vi "Auto Encoder Steering.vi"(8 "Backward":bool, 9 "Gyro Angle":dbl, 11 "Angle setpoint":dbl) -> (1 "Steering":dbl, 3 "Angle error":dbl)   [LabVIEW 2013]
uses:
  Robot Global Data.vi
  <vilib>/addons/control/pid/pid.llb/PID (DBL).vi
  <vilib>/addons/control/pid/NI_PID_pid.lvlib
panel:
  in  "Auto/Control/Steer Limit":dbl=0.7 caption="Turning Limit"
  out "Auto/Output/Gyro Error":dbl caption="Output"
  in  "Auto/Control/Drift Correction Backward Gryo":dbl=0.08 caption="Steering Power"
  in  "Auto/Control/Drift Correction Forward Gryo":dbl=-0.08 caption="Steering Power"
  in  "Auto/Control/Drift Correction Backward":dbl=0.007 caption="Steering Power"
  in  "Auto/Control/Gryo Steering":bool=TRUE caption="Gryo Steering"
  out "Auto/Output/Steering":dbl caption="Output"
  in  "Auto/Control/Drift Correction Forward":dbl=0.007 caption="Steering Power"
  out "Auto/Output/Encoder Error":dbl caption="Output"
  out "Steering Output Graph":dbl(graph)
  in  "Left Dist":dbl
  in  "Right Dist":dbl
  out "Error":dbl(graph)
  # "Steering Power"
  # "Encoder"
  # "Gyro"
  # "Error"
  # "Forward"
  # "Backward"
  # "Drive X-Axis power\nper 1 encoder unit\ndifference L/R"
  # "DISABLED -->"
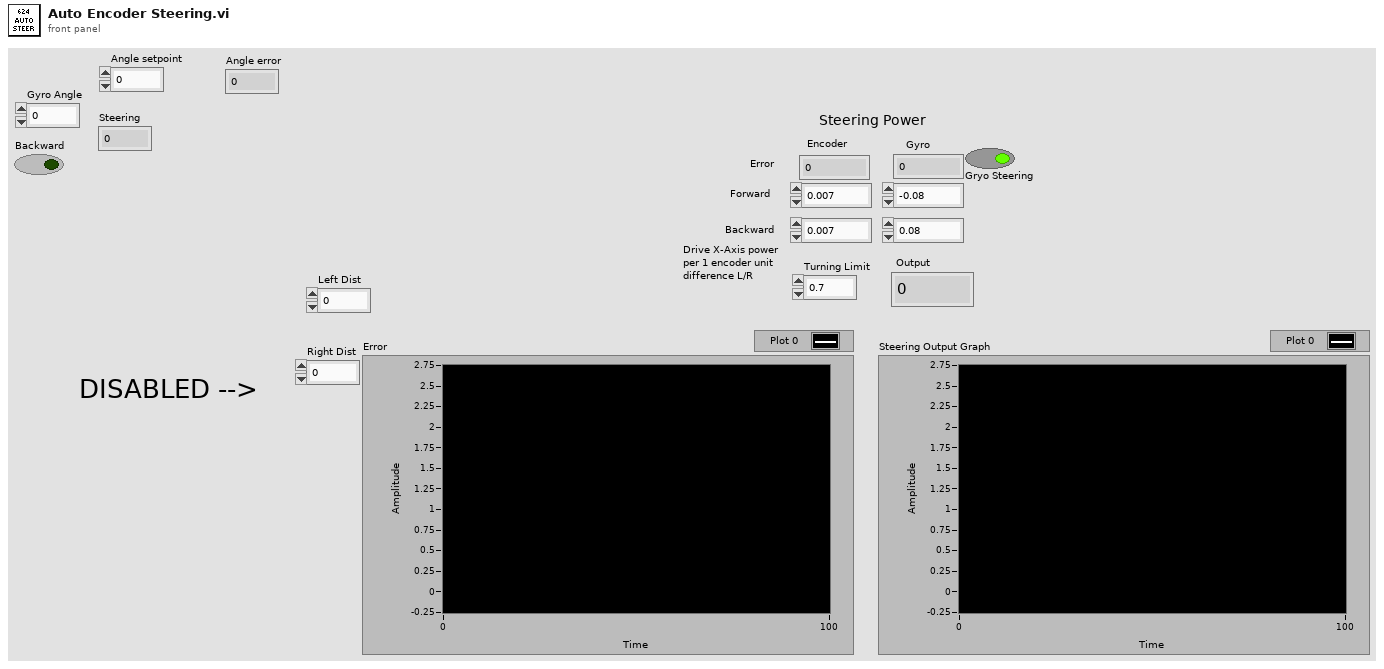
[diagram p1: front panel]
types:
  T1 = typedef "Encoder Values.ctl" = cluster{"Left Dist":dbl, "Left Speed":dbl, "Right Dist":dbl, "Right Speed":dbl, "Left Ticks":dbl, "Right Ticks":dbl, "Avg Distance":dbl, "Avg Speed":dbl}
  T2 = typedef "UDP Dashboard Packet.ctl" = cluster{"Feed Angle":dbl, "Neutral Angle":dbl, "Autonomous Setpoints":T3, "Auto Shift":T4, "Elevator Angle Offset":dbl, "Potentiometer Angle":cluster{"Pot M":dbl, "Pot B":dbl}, "Shoot Setpoints":cluster{"Vision":T5, "Back Corner":T5, "Front":T5, "Front Corner":T5, "Half Court":T5, "Full Court":T5, "Pyramid":T5}, "Halo Drive":T6, "Auto Speed Constants":T7, "Shooting Delays":cluster{"Unjam On":dbl, "Unjam Off":dbl, "Flipper On":dbl, "Flipper Off":dbl, "Hopper Up":dbl}, "Left Roller Pwr":dbl, "Right Roller Pwr":dbl, "Elevator PID Gains":cluster{"proportional gain (Kc)":dbl, "integral time (Ti, min)":dbl, "derivative time (Td, min)":dbl}, "Elevator PID Output Range":cluster{"output high":dbl, "output low":dbl}, "Elevator Angle Tolerance":dbl, "Toggle Ears Delay":dbl, "Toggle Ears Distance":dbl, "Unjam Servo Angle":dbl, "Auton Steer PID gains":cluster{"proportional gain (Kc)":dbl, "integral time (Ti, min)":dbl, "derivative time (Td, min)":dbl}, "Auton Steer output range":cluster{"output high":dbl, "output low":dbl}, "Auto Reverse Speed":dbl, "Auto Stop Throttle":dbl, "Auto Stop Duration":dbl, "Spin output range":cluster{"output high":dbl, "output low":dbl}, "Spin PID gains":cluster{"proportional gain (Kc)":dbl, "integral time (Ti, min)":dbl, "derivative time (Td, min)":dbl}, "Auto-Center Line":T8, "Auton Distance PID gains Low Gear":cluster{"proportional gain (Kc)":dbl, "integral time (Ti, min)":dbl, "derivative time (Td, min)":dbl}, "Auton Distance output range":cluster{"output high":dbl, "output low":dbl}, "Auton Distance Threshold":dbl, "Auton Velocity Cutoff":dbl, "Auton Distance output range Center Line":cluster{"output high":dbl, "output low":dbl}, "Auton Distance PID gains High Gear":cluster{"proportional gain (Kc)":dbl, "integral time (Ti, min)":dbl, "derivative time (Td, min)":dbl}}
  T3 = typedef "Autonomous Setpoints.ctl" = cluster{"Shoot Angle 1":dbl, "Initial Delay":dbl, "Disc Count 1":dbl, "Shoot Time 1":dbl, "Distance 1":dbl, "Two Disc Distance 1":dbl, "Distance 2":dbl, "Two Disc Distance 2":dbl, "Distance 3":dbl, "Two Disc Distance 3":dbl, "Shoot Angle 3":dbl, "Disc Count 3":dbl, "Shoot Time 3":dbl, "Distance 4":dbl, "Two Disc Distance 4":dbl, "Low Gear":bool, "Shoot 1 Post Delay":dbl}
  T4 = typedef "Auto Shift Settings.ctl" = cluster{"Enabled":bool, "Upshift Speed":dbl, "Downshift Speed":dbl, "Upshift Throttle":dbl, "Turn Power Diff":dbl, "Motor Limit":dbl, "Encoder Limit":dbl}
  T5 = typedef "Shoot Profile.ctl" = cluster{"Pre RPM":dbl, "Main RPM":dbl, "Angle":dbl}
  T6 = typedef "Halo Drive.ctl" = cluster{"Gains":cluster{"Quickturn_Sens_Low":dbl, "Quickturn_Sens_High":dbl, "Speedturn_Sens_Low":dbl, "Speedturn_Sens_High":dbl}, "QuickTurn Const":dbl, "Loading Throttle Limit":dbl}
  T7 = typedef "Auto Speed Constants.ctl" = cluster{"Slowing Distance":dbl, "High Speed":dbl, "Rampup Time":dbl, "Low Speed":dbl, "High Speed (Reverse)":dbl}
  T8 = typedef "Autonomous Center Line Setpoints.ctl" = cluster{"Arc Turn x-axis":dbl, "Arc Turn y-axis":dbl, "Arc Turn Distance":dbl, "Distance 1":dbl, "Two Disc Distance 1":dbl, "Distance 2":dbl, "Two Disc Distance 2":dbl, "Spin Angle":dbl, "Spin Angle tolerance":dbl, "Spin y-axis":dbl, "Spin Distance":dbl, "Center Line Enabled":bool, "Distance 3":dbl, "Two Disc Distance 3":dbl, "Spin Angle 2":dbl, "Spin Angle tolerance 2":dbl, "Spin y-axis 2":dbl, "Spin Distance 2":dbl, "Shoot Angle 1":dbl, "Disc Count 1":dbl, "Shoot Time 1":dbl, "Shoot Angle 3":dbl, "Disc Count 3":dbl, "Shoot Time 3":dbl, "Low Gear":bool}
  T9 = cluster{"proportional gain (Kc)":dbl, "integral time (Ti, min)":dbl, "derivative time (Td, min)":dbl}
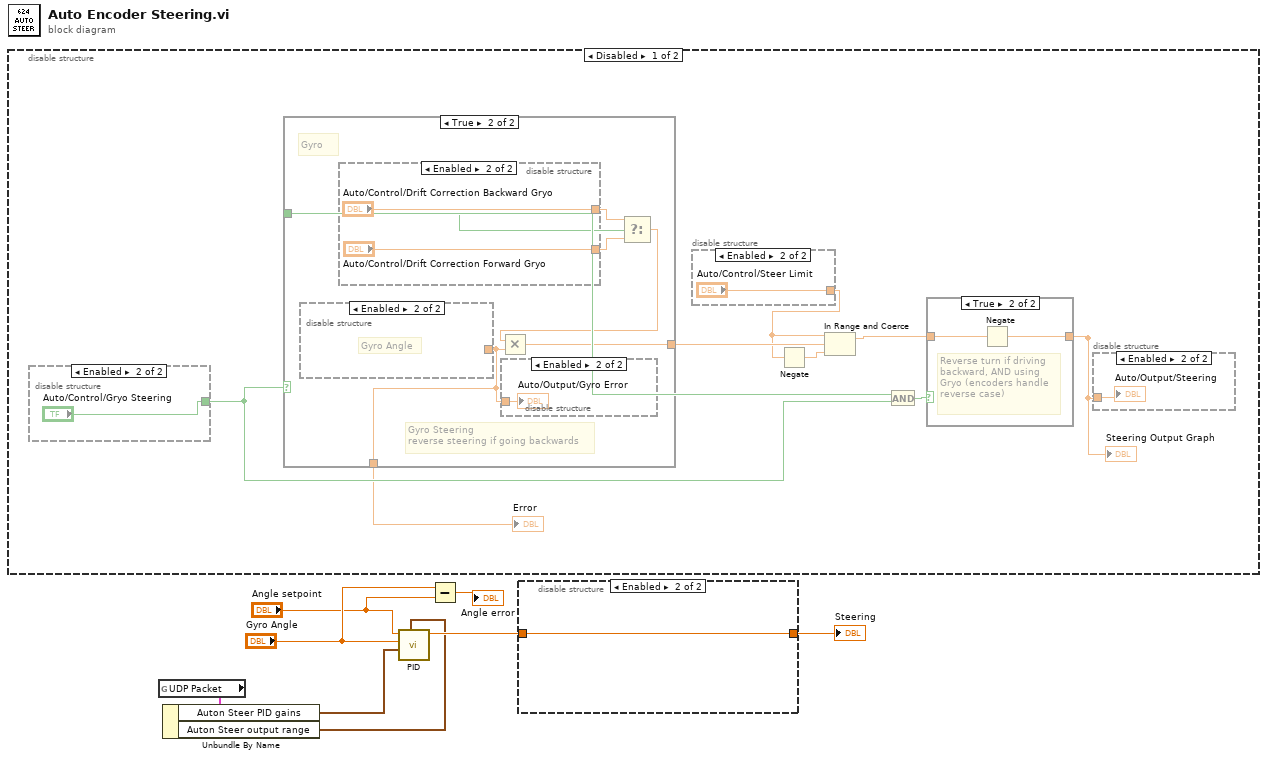
[diagram p0: block diagram]
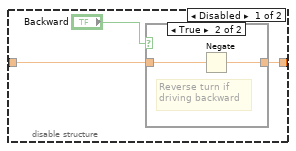
[diagram p2: hidden frame]
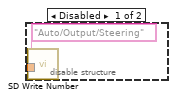
[diagram p4: hidden frame]
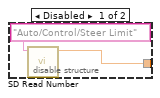
[diagram p5: hidden frame]
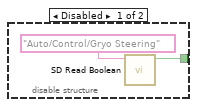
[diagram p6: hidden frame]
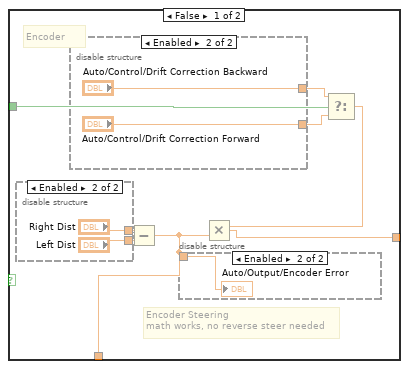
[diagram p7: hidden frame]
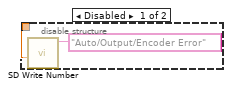
[diagram p8: hidden frame]
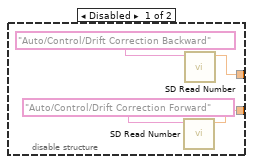
[diagram p9: hidden frame]
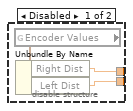
[diagram p10: hidden frame]
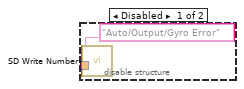
[diagram p11: hidden frame]
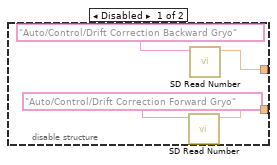
[diagram p12: hidden frame]
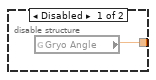
[diagram p13: hidden frame]
diagram:
  n1 = disable-structure shown="Disabled" {
    frame Disabled {
      n2 = disable-structure shown="Enabled" {
        disable-tunnel: [w24 "Auto/Control/Gryo Steering"] -> w13
        frame Disabled {
          n3 = call <vilib>:"SD Read Boolean.vi"("Name"="Auto/Control/Gryo Steering") -> ("Boolean"=w24:bool)  [unwired: 8 in, 2 out]
        }
        frame Enabled {
        }
      }
      n4 = case shown="True" w13 {
        tunnel: [w31 w50] -> w16
        tunnel: [w30 w51] -> w12
        tunnel: [w29 w49] -> w10
        frame False {
          # "Encoder"
          # "Encoder Steering\nmath works, no reverse steer needed"
          n5 = disable-structure shown="Enabled" {
            disable-tunnel: [w45 "Right Dist"] -> w28
            disable-tunnel: [w44 "Left Dist"] -> w27
            frame Disabled {
              n6 = global read "Robot Global Data.vi" "Encoder Values"() -> (w46:T1)
              n7 = Unbundle By Name(w46) -> ("Right Dist"=w45:dbl, "Left Dist"=w44:dbl)
            }
            frame Enabled {
            }
          }
          n8 = disable-structure shown="Enabled" {
            disable-tunnel: [w41 "Auto/Control/Drift Correction Forward"] -> w34
            disable-tunnel: [w40 "Auto/Control/Drift Correction Backward"] -> w33
            frame Disabled {
              n9 = call <vilib>:"SD Read Number.vi"("Name"="Auto/Control/Drift Correction Forward") -> ("Numeric"=w41:dbl)  [unwired: 8 in, 2 out]
              n10 = call <vilib>:"SD Read Number.vi"("Name"="Auto/Control/Drift Correction Backward") -> ("Numeric"=w40:dbl)  [unwired: 8 in, 2 out]
            }
            frame Enabled {
            }
          }
          n11 = Subtract(x=w28, y=w27) -> (x-y=w29:dbl)
          n12 = disable-structure shown="Enabled" {
            disable-tunnel: w29 -> [w35 w37]
            frame Disabled {
              n13 = call <vilib>:"SD Write Number.vi"("Numeric"=w35, "Name"="Auto/Output/Encoder Error") -> ()  [unwired: 8 in, 2 out]
            }
            frame Enabled {
              "Auto/Output/Encoder Error" <- w37
            }
          }
          n14 = Select(t=w33, s=w30, f=w34) -> (s? t:f=w32:dbl)
          n15 = Multiply(x=w32, y=w29) -> (x*y=w31:dbl)
        }
        frame True {
          # "Gyro"
          # "Gyro Steering\nreverse steering if going backwards"
          n16 = disable-structure shown="Enabled" {
            disable-tunnel: [w64 w65] -> w49
            frame Disabled {
              n17 = global read "Robot Global Data.vi" "Gryo Angle"() -> (w64:dbl)
            }
            frame Enabled {
              # "Gyro Angle"
            }
          }
          n18 = disable-structure shown="Enabled" {
            disable-tunnel: [w61 "Auto/Control/Drift Correction Forward Gryo"] -> w54
            disable-tunnel: [w60 "Auto/Control/Drift Correction Backward Gryo"] -> w53
            frame Disabled {
              n19 = call <vilib>:"SD Read Number.vi"("Name"="Auto/Control/Drift Correction Forward Gryo") -> ("Numeric"=w61:dbl)  [unwired: 8 in, 2 out]
              n20 = call <vilib>:"SD Read Number.vi"("Name"="Auto/Control/Drift Correction Backward Gryo") -> ("Numeric"=w60:dbl)  [unwired: 8 in, 2 out]
            }
            frame Enabled {
            }
          }
          n21 = disable-structure shown="Enabled" {
            disable-tunnel: w49 -> [w55 w57]
            frame Disabled {
              n22 = call <vilib>:"SD Write Number.vi"("Numeric"=w55, "Name"="Auto/Output/Gyro Error") -> ()  [unwired: 8 in, 2 out]
            }
            frame Enabled {
              "Auto/Output/Gyro Error" <- w57
            }
          }
          n23 = Select(t=w53, s=w51, f=w54) -> (s? t:f=w52:dbl)
          n24 = Multiply(x=w52, y=w49) -> (x*y=w50:dbl)
        }
      }
      "Error" <- w10
      n25 = disable-structure shown="Enabled" {
        disable-tunnel: [w21 "Auto/Control/Steer Limit"] -> w14
        frame Disabled {
          n26 = call <vilib>:"SD Read Number.vi"("Name"="Auto/Control/Steer Limit") -> ("Numeric"=w21:dbl)  [unwired: 8 in, 2 out]
        }
        frame Enabled {
        }
      }
      n27 = Negate(x=w14) -> (-x=w15:dbl)
      n28 = In Range and Coerce(upper limit=w14, x=w16, lower limit=w15) -> (coerced(x)=w17:dbl)  [unwired: 1 out]
      n29 = And(x=w12, y=w13) -> (x .and. y?=w11:bool)
      n30 = case shown="True" w11 {
        tunnel: w17 -> [w66 w68]
        tunnel: [w66 w67] -> w9
        frame False {
        }
        frame True {
          # "Reverse turn if driving\nbackward, AND using\nGryo (encoders handle\nreverse case)"
          n31 = Negate(x=w68) -> (-x=w67:dbl)
        }
      }
      "Steering Output Graph" <- w9
      n32 = disable-structure shown="Enabled" {
        disable-tunnel: w9 -> [w18 w20]
        frame Disabled {
          n33 = call <vilib>:"SD Write Number.vi"("Numeric"=w18, "Name"="Auto/Output/Steering") -> ()  [unwired: 8 in, 2 out]
        }
        frame Enabled {
          "Auto/Output/Steering" <- w20
        }
      }
    }
    frame Enabled {
    }
  }
  n34 = global read "Robot Global Data.vi" "UDP Packet"() -> (w6:T2)
  n35 = Unbundle By Name(w6) -> ("Auton Steer PID gains"=w4:T9, "Auton Steer output range"=w5:cluster{"output high":dbl, "output low":dbl})
  n36 = call-poly <vilib>:"PID.vi"("output range"=w5, "PID gains"=w4, "process variable"="Gyro Angle", "setpoint"="Angle setpoint") -> ("output"=w8:dbl)  [unwired: 6 in, 1 out]
  n37 = Subtract(x="Gyro Angle", y="Angle setpoint") -> (x-y=→"Angle error":dbl)
  n38 = disable-structure shown="Enabled" {
    disable-tunnel: w8 -> [w71 w75]
    disable-tunnel: [w70 w75] -> w7
    frame Disabled {
      n39 = case shown="True" "Backward" {
        tunnel: w71 -> [w72 w74]
        tunnel: [w72 w73] -> w70
        frame False {
        }
        frame True {
          # "Reverse turn if\ndriving backward"
          n40 = Negate(x=w74) -> (-x=w73:dbl)
        }
      }
    }
    frame Enabled {
    }
  }
  "Steering" <- w7
